vi "Voltage_current_hysteresis.vi"() -> ()   [LabVIEW 2017]
uses:
  <instrlib>/niDCPower/nidcpower.llb/niDCPower Source Mode.ctl
  <instrlib>/niDCPower/nidcpower.llb/niDCPower Wait For Event - Event.ctl
  <instrlib>/niDCPower/nidcpower.llb/niDCPower Output Function.ctl
  <vilib>/Utility/error.llb/DialogType.ctl
  <instrlib>/niDCPower/nidcpower.llb/niDCPower Sense.ctl
panel:
  in  "time to wait for field, ms":u32
  out "ResistanceCurrent":T1(graph)={"voltage measurements"=[-1.607620338425132e-08, -1.56894905880665e-08, -1.2761522274095711e-08, -1.2006511576782489e-08, -1.1675043465770316e-08, -1.1527724305315567e-08, -1.2006511576782489e-08, -1.1251500879472655e-08, -1.0920032768457094e-08, -1.0422830601933752e-08, -9.39159647877084e-09, -7.365958022568023e-09, -7.586936763245063e-09, -4.603723764105014e-09, -2.5228406227295478e-09, -1.970393771036946e-09, -2.596500202955228e-09, -4.143351387694513e-09, -3.4804151656633907e-09, -2.301861882052507e-09, -2.0808831413754664e-09, -1.2153830737237237e-09, -1.4363618144007644e-09, -5.156170615831497e-10, 1.988808666093366e-09, 3.3883406903779023e-09, 3.6645641162275913e-09, 4.198596072863773e-09, 4.327500338258713e-09, 4.290670548142485e-09, 4.1249364926347046e-09, 3.867127961844824e-09, 3.7198088013968515e-09, 4.437989708597234e-09, 4.879947189947927e-09, 5.91118131310745e-09, 7.771085713805876e-09, 8.581341096288358e-09, 9.33635179360158e-09, 9.704649694729982e-09, 9.465256058996521e-09, 9.11537305292454e-09, 8.8943943122475e-09, 8.562926201231938e-09, 8.857564522134659e-09, 9.09695815786812e-09, 1.0036117805745543e-08, 1.0791128503058765e-08, 1.254054353341867e-08, 1.3442873391183253e-08, 1.3940075557706595e-08, 1.4271543668722156e-08, 1.3645437236803874e-08, 1.3663852131860294e-08, 1.3166649965336952e-08, 1.2761522274095711e-08, 1.3258724440619053e-08, 1.3074575490054852e-08, 1.3976905347819435e-08, 1.5026554366035378e-08, 1.6610235340887503e-08, 1.812025673551056e-08, 1.869111848226297e-08, 1.878319295754168e-08, 1.8249161000908888e-08, 1.7623054568990606e-08, 1.7015363032128744e-08, 1.6352426810097622e-08, 1.6960118346959484e-08, 1.7659884359103446e-08, 1.8028182260231847e-08, 1.926198022901199e-08, 2.0900905889029988e-08, 2.1527012320951658e-08, 2.161908679623037e-08, 2.0919320784086408e-08, 2.0643097358243495e-08, 2.121395910498913e-08, 2.125078889510197e-08, 2.0422118617563067e-08, 2.0164310086776574e-08, 2.0256384562055286e-08, 2.0698342043412756e-08, 2.119554420993271e-08, 2.3276427351308175e-08, 2.493376790638598e-08, 2.6093906294940444e-08, 2.5780853078981303e-08, 2.509950196189376e-08, 2.493376790638598e-08, 2.3497406091985216e-08, 2.3681555042549417e-08, 2.465754448053968e-08, 2.5817682869094143e-08, 2.6149150980109704e-08, 2.808271496103381e-08, 2.9169193769362594e-08, 3.071604495410188e-08], "current measurements"=[]} caption="Current (Amps) vs Voltage (Volts)"
  in  "Measurement type":bool=TRUE
  in  "Number of loops":i32 min=0 step=1
  in  "Field, Oe":dbl min=-4000.0 max=4000.0
  in  "Source Delay (Sec)":dbl=0.005
  in  "Current Limit":dbl=0.001 caption="Current Limit, A"
  out "VoltageCurrent":T1(graph)={"voltage measurements"=[-0.0999994140167501, -0.09797954272446788, -0.09595969680554058, -0.09393895436140587, -0.09191882933557437, -0.08989828987827908, -0.08787949272468874, -0.08585836122244515, -0.0838384307256681, -0.08181749375247895, -0.07979821450514502, -0.07777748897658025, -0.07575678036358545, -0.07373644389312957, -0.07171707161016089, -0.0696969127531895, -0.06767759121693066, -0.06565663732817158, -0.06363639389335043, -0.06161570219592557, -0.05959569557908372, -0.05757547751761751, -0.055555496274130596, -0.053535980208817335, -0.051515043235628194, -0.04949432616484841, -0.04747449716149106, -0.04545444825572434, -0.043433604318169935, -0.041414426564255695, -0.039394910498942434, -0.03737443870392695, -0.03535368780200727, -0.03333309759800211, -0.03131324322128984, -0.029293016702038634, -0.027272646400442857, -0.02525307958841974, -0.023232929189233323, -0.02121263500770232, -0.01919163037223337, -0.017171539177541773, -0.01515202311222852, -0.013130993103404641, -0.011111764602780553, -0.009091707239228862, -0.007070880217244401, -0.00505033230216413, -0.00302927691998533, -0.0010099722992964588, 0.0010099920286205004, 0.0030304215347111132, 0.005050901787511579, 0.007071458160376826, 0.00909073740771077, 0.01111070173562773, 0.013130826761459224, 0.015152110503832363, 0.0171721171206742, 0.019191675474912337, 0.021211402984849984, 0.023232280753544297, 0.025251856023352386, 0.02727315668129547, 0.029293044889147656, 0.03131237488319145, 0.03333345563872518, 0.035354045842730324, 0.03737311364543988, 0.03939347548925069, 0.04141445475136472, 0.04343490117302528, 0.045454941621007015, 0.04747478753993432, 0.04949473495228133, 0.05151533361407146, 0.053535441724333, 0.05555493241629132, 0.05757563257150116, 0.05959562227277304, 0.061616085610003556, 0.06363632058703973, 0.06565705457338947, 0.06767657063870272, 0.0696969409402985, 0.07171769184221818, 0.07373800293931915, 0.07575691004411417, 0.07777853209788632, 0.07979770985180056, 0.08181830851359068, 0.08383795990346354, 0.08585846552961894, 0.08787892040906448, 0.08989940911964991, 0.09191923812300727, 0.09393979449587252, 0.09595983494385425, 0.09797928334688771, 0.09999958598620369], "current measurements"=[-1.4768745835245497e-08, -1.607620338425132e-08, -1.56894905880665e-08, -1.2761522274095711e-08, -1.2006511576782489e-08, -1.1675043465770316e-08, -1.1527724305315567e-08, -1.2006511576782489e-08, -1.1251500879472655e-08, -1.0920032768457094e-08, -1.0422830601933752e-08, -9.39159647877084e-09, -7.365958022568023e-09, -7.586936763245063e-09, -4.603723764105014e-09, -2.5228406227295478e-09, -1.970393771036946e-09, -2.596500202955228e-09, -4.143351387694513e-09, -3.4804151656633907e-09, -2.301861882052507e-09, -2.0808831413754664e-09, -1.2153830737237237e-09, -1.4363618144007644e-09, -5.156170615831497e-10, 1.988808666093366e-09, 3.3883406903779023e-09, 3.6645641162275913e-09, 4.198596072863773e-09, 4.327500338258713e-09, 4.290670548142485e-09, 4.1249364926347046e-09, 3.867127961844824e-09, 3.7198088013968515e-09, 4.437989708597234e-09, 4.879947189947927e-09, 5.91118131310745e-09, 7.771085713805876e-09, 8.581341096288358e-09, 9.33635179360158e-09, 9.704649694729982e-09, 9.465256058996521e-09, 9.11537305292454e-09, 8.8943943122475e-09, 8.562926201231938e-09, 8.857564522134659e-09, 9.09695815786812e-09, 1.0036117805745543e-08, 1.0791128503058765e-08, 1.254054353341867e-08, 1.3442873391183253e-08, 1.3940075557706595e-08, 1.4271543668722156e-08, 1.3645437236803874e-08, 1.3663852131860294e-08, 1.3166649965336952e-08, 1.2761522274095711e-08, 1.3258724440619053e-08, 1.3074575490054852e-08, 1.3976905347819435e-08, 1.5026554366035378e-08, 1.6610235340887503e-08, 1.812025673551056e-08, 1.869111848226297e-08, 1.878319295754168e-08, 1.8249161000908888e-08, 1.7623054568990606e-08, 1.7015363032128744e-08, 1.6352426810097622e-08, 1.6960118346959484e-08, 1.7659884359103446e-08, 1.8028182260231847e-08, 1.926198022901199e-08, 2.0900905889029988e-08, 2.1527012320951658e-08, 2.161908679623037e-08, 2.0919320784086408e-08, 2.0643097358243495e-08, 2.121395910498913e-08, 2.125078889510197e-08, 2.0422118617563067e-08, 2.0164310086776574e-08, 2.0256384562055286e-08, 2.0698342043412756e-08, 2.119554420993271e-08, 2.3276427351308175e-08, 2.493376790638598e-08, 2.6093906294940444e-08, 2.5780853078981303e-08, 2.509950196189376e-08, 2.493376790638598e-08, 2.3497406091985216e-08, 2.3681555042549417e-08, 2.465754448053968e-08, 2.5817682869094143e-08, 2.6149150980109704e-08, 2.808271496103381e-08, 2.9169193769362594e-08, 3.071604495410188e-08, 3.10106832750046e-08]} caption="Current (Amps) vs Voltage (Volts)"
  in  "Voltage Level Stop":dbl=0.1 caption="Voltage Level Stop, V"
  in  "Voltage Level Start":dbl=-0.1 caption="Voltage Level Start, V"
  in  "Points":i32=100 min=1
  # "2-points"
  # "4-points"
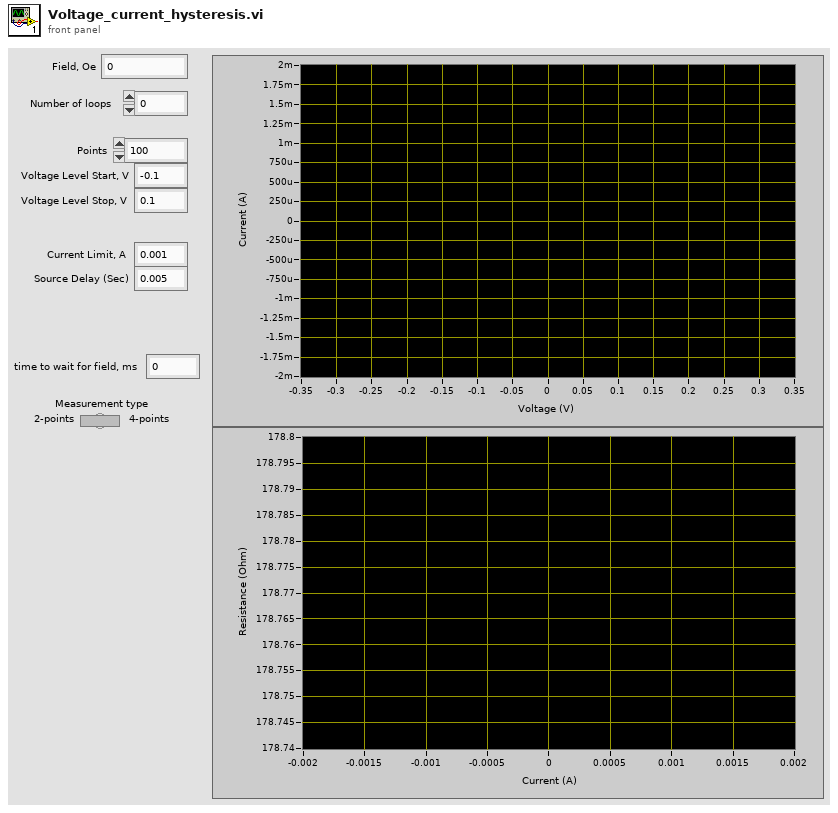
[diagram p1: front panel]
types:
  T1 = cluster{"voltage measurements":dbl[], "current measurements":dbl[]}
  T2 = typedef "DialogType.ctl" = u16
  T3 = typedef "niDCPower Output Function.ctl" = i32
  T4 = typedef "niDCPower Wait For Event - Event.ctl" = i32
  T5 = typedef "niDCPower Source Mode.ctl" = i32
  T6 = typedef "niDCPower Sense.ctl" = i32
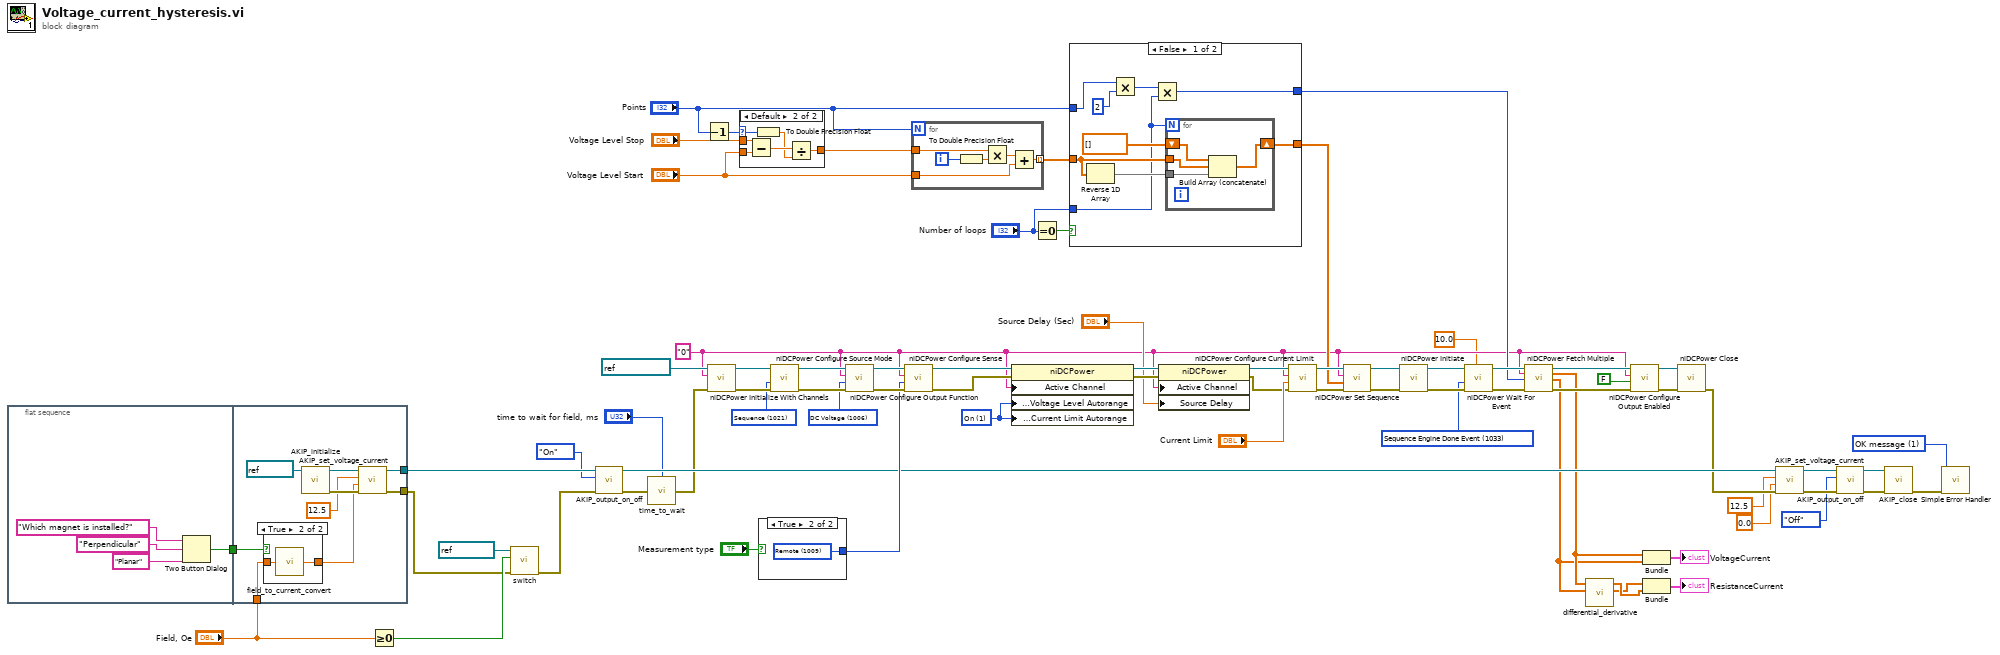
[diagram p0: block diagram]
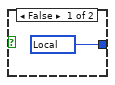
[diagram p2: hidden frame]
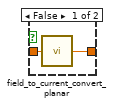
[diagram p4: hidden frame]
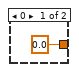
[diagram p5: hidden frame]
diagram:
  w13 = T2 1 items=["no dialog", "OK message", "continue or stop message", "OK message + warnings", "continue/stop + warnings"] ("type of dialog (OK msg:1)")
  w23 = "0" ("SMU Channel Name")
  w43 = T3 1006 items=["DC Voltage"=1006, "DC Current"=1007, "Pulse Voltage"=1049, "Pulse Current"=1050] ("output function")
  w54 = T4 1033 items=["Source Complete Event"=1030, "Measure Complete Event"=1031, "Sequence Iteration Complete Event"=1032, "Sequence Engine Done Event"=1033] ("event")
  w62 = T5 1021 items=["Single Point"=1020, "Sequence"=1021] ("source mode")
  w44 = 1 items=["Off", "On"] ("DC Voltage:Voltage Level Autorange")
  n1 = flat-sequence {
    tunnel: [w75] -> w41
    tunnel: w41 -> [w83]
    tunnel: "Field, Oe" -> [w82]
    tunnel: [w80] -> w36
    tunnel: [w79] -> w40
    frame #0 {
      n2 = Two Button Dialog(message="Which magnet is installed?", 1:"Planar" ("F button name (\"Cancel\")"), 2:"Perpendicular" ("T button name (\"OK\")")) -> (T button?=w75:bool)
    }
    frame #1 {
      n3 = case shown="True" w83 {
        tunnel: w82 -> [w89 w91]
        tunnel: [w88 w90] -> w81
        frame False {
          n4 = call "field_to_current_convert_planar.vi"("Field, Oe"=w89) -> ("Current, A"=w88:dbl)
        }
        frame True {
          n5 = call "field_to_current_convert.vi"("Field, Oe"=w91) -> ("Current, A"=w90:dbl)
        }
      }
      n6 = call "AKIP_initialize.vi"("VISA Refnum in"=refnum<visa-resource-name> "AKIP") -> ("error out"=w87:errorcluster, "VISA Refnum out"=w86:refnum<visa-resource-name>)  [unwired: 9 in]
      n7 = call "AKIP_set_voltage_current.vi"("error in (no error)"=w87, "Current"=w81, "Voltage"=12.5, "VISA resource name (in)"=w86) -> ("error out"=w80:errorcluster, "VISA resource name (out)"=w79:refnum<visa-resource-name>)  [unwired: 6 in]
    }
  }
  n8 = Greater Or Equal To 0?(x="Field, Oe") -> (x >= 0?=w37:bool)
  n9 = call "switch.vi"("error in (no error)"=w36, "Positive?"=w37, "Switch port (in)"=refnum<visa-resource-name> "Switch") -> ("error out"=w35:errorcluster)  [unwired: 7 in, 1 out]
  n10 = call "AKIP_output_on_off.vi"("error in (no error)"=w35, "Enum"=enum16{"On", "Off"}."On", "VISA Refnum in"=w40) -> ("error out"=w9:errorcluster, "VISA Refnum out"=w20:refnum<visa-resource-name>)  [unwired: 7 in]
  n11 = call "time_to_wait.vi"("error in (no error)"=w9, "milliseconds to wait"="time to wait for field, ms") -> ("error out"=w8:errorcluster)
  n12 = Decrement(x="Points") -> (x-1=w71:i32)
  n13 = call <instrlib>:"niDCPower Initialize With Channels.vi"("error in (no error)"=w8, "channels"=w23, "resource name"=refnum<k15> "SMU4137") -> ("error out"=w66:errorcluster, "instrument handle out"=w63:refnum<k15>)  [unwired: 2 in, 5 out]
  n14 = case shown="Default" w71 {
    selector: w71 -> [_ w93]
    tunnel: "Voltage Level Stop" -> [_ w98]
    tunnel: [0.0 w96] -> w70
    tunnel: "Voltage Level Start" -> [_ w94]
    frame 0 {
    }
    frame Default {
      n15 = Subtract(x=w98, y=w94) -> (x-y=w97:dbl)
      n16 = To Double Precision Float(number=w93) -> (double precision float=w95:dbl)
      n17 = Divide(x=w97, y=w95) -> (x/y=w96:dbl)
    }
  }
  n18 = case shown="True" "Measurement type" {
    tunnel: [w99 w100] -> w21
    frame False {
      w99 = T6 1008 items=["Local"=1008, "Remote"=1009] ("sense")
    }
    frame True {
      w100 = T6 1009 items=["Local"=1008, "Remote"=1009] ("sense")
    }
  }
  n19 = call <instrlib>:"niDCPower Configure Source Mode.vi"("error in (no error)"=w66, "source mode"=w62, "instrument handle"=w63) -> ("error out"=w65:errorcluster, "instrument handle out"=w64:refnum<k15>)  [unwired: 7 out]
  n20 = call <instrlib>:"niDCPower Configure Output Function.vi"("error in (no error)"=w65, "output function"=w43, "channel name"=w23, "instrument handle"=w64) -> ("error out"=w26:errorcluster, "instrument handle out"=w27:refnum<k15>)  [unwired: 6 out]
  n21 = call <instrlib>:"niDCPower Configure Sense.vi"("error in (no error)"=w26, "sense"=w21, "channel name"=w23, "instrument handle"=w27) -> ("error out"=w24:errorcluster, "instrument handle out"=w25:refnum<k15>)  [unwired: 6 in]
  n22 = for {
    N: "Points" -> [_]
    tunnel: w70 -> [w106]
    tunnel: "Voltage Level Start" -> [w103]
    tunnel: [w101] -> w33 mode=indexing
    i -> [w105]
    n23 = To Double Precision Float(number=w105) -> (double precision float=w102:dbl)
    n24 = Multiply(x=w106, y=w102) -> (x*y=w104:dbl)
    n25 = Add(x=w104, y=w103) -> (x+y=w101:dbl)
  }
  n26 = property class="niDCPower"(reference=w25, error in=w24, "Active Channel"=w23, "Source:DC Voltage:Voltage Level Autorange"=w44, "Source:DC Voltage:Current Limit Autorange"=w44) -> (reference out=w61:refnum<k15>, error out=w60:errorcluster)
  n27 = Equal To 0?(x="Number of loops") -> (x = 0?=w31:bool)
  n28 = case shown="False" w31 {
    tunnel: w33 -> [w115 w121]
    tunnel: "Points" -> [w111 w120]
    tunnel: [w112 w121] -> w30
    tunnel: [w107 w120] -> w29
    tunnel: "Number of loops" -> [w108 _]
    frame False {
      n29 = Reverse 1D Array(array=w115) -> (reversed array=w114:dbl[])
      n30 = Multiply(x=w111, y=2) -> (x*y=w109:i32)
      n31 = Multiply(x=w109, y=w108) -> (x*y=w107:i32)
      n32 = for {
        N: w108 -> [_]
        shift-right: [w116] -> w112
        shift-left: dbl[] [] -> [w117]
        tunnel: w115 -> [w118]
        tunnel: w114 -> [w119]
        n33 = Build Array (concatenate)(w117, w118, w119) -> (w116:dbl[])
      }
    }
    frame True {
    }
  }
  n34 = property class="niDCPower"(reference=w61, error in=w60, "Active Channel"=w23, "Source Delay"="Source Delay (Sec)") -> (reference out=w59:refnum<k15>, error out=w58:errorcluster)
  n35 = call <instrlib>:"niDCPower Configure Current Limit.vi"("error in (no error)"=w58, "current limit"="Current Limit", "channel name"=w23, "instrument handle"=w59) -> ("error out"=w68:errorcluster, "instrument handle out"=w67:refnum<k15>)  [unwired: 6 out]
  n36 = call <instrlib>:"niDCPower Set Sequence.vi"("error in (no error)"=w68, "values"=w30, "channel name"=w23, "instrument handle"=w67) -> ("error out"=w47:errorcluster, "instrument handle out"=w46:refnum<k15>)  [unwired: 1 in, 5 out]
  n37 = call <instrlib>:"niDCPower Initiate.vi"("error in (no error)"=w47, "instrument handle"=w46) -> ("error out"=w56:errorcluster, "instrument handle out"=w49:refnum<k15>)  [unwired: 8 out]
  n38 = call <instrlib>:"niDCPower Wait For Event.vi"("timeout (sec)"=10.0, "error in (no error)"=w56, "event"=w54, "instrument handle"=w49) -> ("error out"=w55:errorcluster, "instrument handle out"=w48:refnum<k15>)  [unwired: 6 out]
  n39 = call <instrlib>:"niDCPower Fetch Multiple.vi"("instrument handle"=w48, "channel name"=w23, "count (1)"=w29, "error in (no error)"=w55) -> ("instrument handle out"=w50:refnum<k15>, "voltage measurements"=w7:dbl[], "current measurements"=w5:dbl[], "error out"=w52:errorcluster)  [unwired: 1 in, 7 out]
  n40 = call "differential_derivative.vi"("X"=w5, "Y"=w7) -> ("X"=w2:dbl[], "dY/dX"=w3:dbl[])  [unwired: 8 in]
  n41 = call <instrlib>:"niDCPower Configure Output Enabled.vi"("error in (no error)"=w52, "output enabled"=FALSE, "channel name"=w23, "instrument handle"=w50) -> ("error out"=w51:errorcluster, "instrument handle out"=w57:refnum<k15>)  [unwired: 6 out]
  n42 = Bundle("voltage measurements"=w7, "current measurements"=w5) -> (→"VoltageCurrent":T1)  [unwired: 1 out]
  n43 = Bundle("X"=w2, "dY/dX"=w3) -> (→"ResistanceCurrent":cluster{"X":dbl[], "dY/dX":dbl[]})  [unwired: 1 out]
  n44 = call <instrlib>:"niDCPower Close.vi"("error in (no error)"=w51, "instrument handle"=w57) -> ("error out"=w17:errorcluster)  [unwired: 9 out]
  n45 = call "AKIP_set_voltage_current.vi"("error in (no error)"=w17, "Current"=0.0, "Voltage"=12.5, "VISA resource name (in)"=w20) -> ("error out"=w18:errorcluster, "VISA resource name (out)"=w19:refnum<visa-resource-name>)  [unwired: 6 in]
  n46 = call "AKIP_output_on_off.vi"("error in (no error)"=w18, "Enum"=enum16{"On", "Off"}."Off", "VISA Refnum in"=w19) -> ("error out"=w11:errorcluster, "VISA Refnum out"=w12:refnum<visa-resource-name>)  [unwired: 7 in]
  n47 = call "AKIP_close.vi"("error in (no error)"=w11, "VISA Refnum in"=w12) -> ("error out"=w10:errorcluster)  [unwired: 8 in, 1 out]
  n48 = call <vilib>:"Simple Error Handler.vi"("type of dialog (OK msg:1)"=w13, "error in (no error)"=w10) -> ()  [unwired: 8 out]
